vi "StaticRegister.vi"() -> ()   [LabVIEW 2020]
panel:
  out "Web":string
  in  "stop":bool
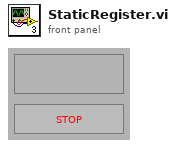
[diagram p1: front panel]
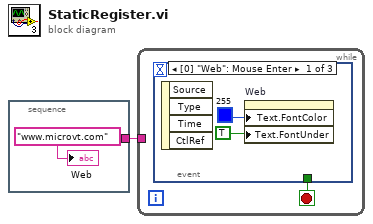
[diagram p0: block diagram]
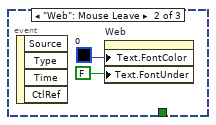
[diagram p2: hidden frame]
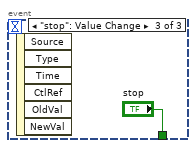
[diagram p3: hidden frame]
diagram:
  n1 = stacked-sequence {
    tunnel: [w2] -> w1
    frame #0 {
      w2 = "www.microvt.com" ("String")
      "Web" <- w2
    }
  }
  n2 = while {
    tunnel: w1 -> [_]
    stop <- w3 stop-if-true
    n3 = event shown="[0] \"Web\": Mouse Enter" {
      selector: _ -> [_ _ _]
      dyn-events: _ -> [_ _ _]
      timeout: _ -> [_ _ _]
      tunnel: [_ _ "stop"] -> w3
      event "Web": Mouse Enter {
        n4 = event-data() -> ()  [unwired: 5 out]
        n5 = property on="Web" class="Str"("Text.FontColor"=u32 255, "Text.FontUnder"=TRUE ("Text.Font:Underline")) -> ()  [unwired: 2 in, 2 out]
      }
      event "Web": Mouse Leave {
        n6 = event-data() -> ()  [unwired: 5 out]
        n7 = property on="Web" class="Str"("Text.FontColor"=u32 0, "Text.FontUnder"=FALSE ("Text.Font:Underline")) -> ()  [unwired: 2 in, 2 out]
      }
      event "stop": Value Change {
        n8 = event-data() -> ()  [unwired: 7 out]
      }
    }
  }
